vi "Read Low Alarm Limit.vi"(8 "error in (no error)":errorcluster, 11 "NT Scalar (Numeric) in":refnum<class "NT Scalar (Numeric).lvclass">) -> (0 "error out":errorcluster, 2 "Low Alarm Limit":variant, 3 "NT Scalar (Numeric) out":refnum<class "NT Scalar (Numeric).lvclass">)   [LabVIEW 2020, in "PV Access.lvlib" / "PV Data.lvlib" / "NT Scalar (Numeric).lvclass"]
uses:
  NT Scalar (Numeric).lvclass
  NT Scalar (Numeric).lvclass/NT Scalar (Numeric).ctl
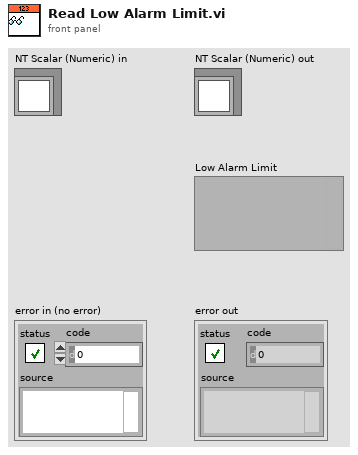
[diagram p1: front panel]
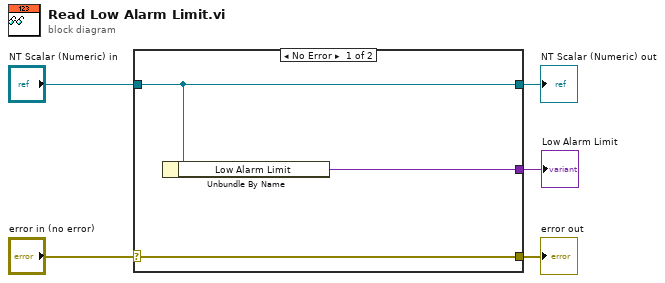
[diagram p0: block diagram]
diagram:
  n1 = case shown="No Error" "error in (no error)" {
    selector: "error in (no error)" -> [w8 w9]
    tunnel: [w8 w9] -> w4
    tunnel: [w7 w10] -> w2
    tunnel: "NT Scalar (Numeric) in" -> [w7 w10]
    tunnel: [w6 _] -> w1
    frame No Error {
      n2 = Unbundle By Name(w7) -> ("Low Alarm Limit"=w6:variant)
    }
    frame Error {
    }
  }
  "error out" <- w4
  "NT Scalar (Numeric) out" <- w2
  "Low Alarm Limit" <- w1
